vi "Focus Set Home.vi"(8 "error in (no error)":errorcluster, 10 "Motor (0:n-1)":i32, 11 "ArduinoFocus in":refnum<class "ArduinoFocus.lvclass">) -> (0 "error out":errorcluster, 3 "ArduinoFocus out":refnum<class "ArduinoFocus.lvclass">)   [LabVIEW 2022 SP3, in "ArduinoFocus.lvclass"]
uses:
  ArduinoFocus.lvclass
  ArduinoFocus.lvclass/ArduinoFocus.ctl
  Motor Control Driver/arduino Motor Control cluster Command.ctl
  Filter Wheel/Filter Wheel Arduino Control/FW Arduino Control.lvclass
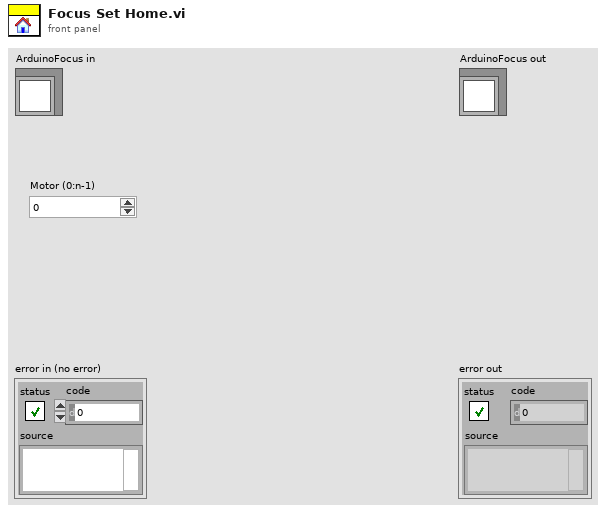
[diagram p1: front panel]
types:
  T1 = typedef "arduino Motor Control cluster Command.ctl" = cluster{"Direction":bool, "NUMBER OF  STEPS":u32, "SPEED STEPS/SEC":u16, "ACC/DECEL STEPS/SEC^2":u16, "EN/DIS?":bool}
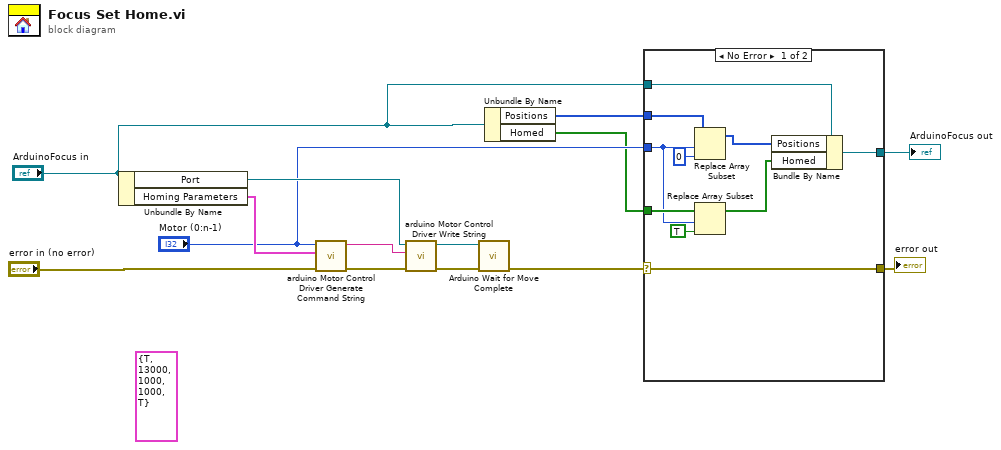
[diagram p0: block diagram]
diagram:
  (unwired) T1 {"Direction"=TRUE, "NUMBER OF  STEPS"=13000, "SPEED STEPS/SEC"=1000, "ACC/DECEL STEPS/SEC^2"=1000, "EN/DIS?"=TRUE} ("Command")
  n1 = Unbundle By Name("ArduinoFocus in") -> ("Port"=w12:refnum<visa-resource-name>, "Homing Parameters"=w8:T1)
  n2 = call "arduino Motor Control Driver Generate Command String.vi"("error in (no error)"="error in (no error)", "Command"=w8, "MOTOR NUMBER"="Motor (0:n-1)") -> ("error out"=w11:errorcluster, "Cmd String"=w13:string)  [unwired: 7 in]
  n3 = call "arduino Motor Control Driver Write String.vi"("error in (no error)"=w11, "String"=w13, "VISA resource name"=w12) -> ("error out"=w9:errorcluster, "VISA resource name out"=w10:refnum<visa-resource-name>)  [unwired: 7 in]
  n4 = call "Arduino Wait for Move Complete.vi"("error in (no error)"=w9, "reference"=w10) -> ("error out"=w5:errorcluster)  [unwired: 6 in, 3 out]
  n5 = Unbundle By Name("ArduinoFocus in") -> ("Positions"=w7:i32[], "Homed"=w4:bool[])
  n6 = case shown="No Error" w5 {
    selector: w5 -> [w15 w25]
    tunnel: w7 -> [w24 _]
    tunnel: "Motor (0:n-1)" -> [w21 _]
    tunnel: w4 -> [w22 _]
    tunnel: "ArduinoFocus in" -> [w19 w26]
    tunnel: [w16 w26] -> w2
    tunnel: [w15 w25] -> w1
    frame No Error {
      n7 = Replace Array Subset(array=w24, new element=0 ("new element/subarray"), index=w21) -> (w18:i32[])
      n8 = Replace Array Subset(array=w22, new element=TRUE ("new element/subarray"), index=w21) -> (w17:bool[])
      n9 = Bundle By Name(cluster=w19, "Positions"=w18, "Homed"=w17) -> (w16:refnum<class "ArduinoFocus.lvclass">)
    }
    frame Error {
    }
  }
  "error out" <- w1
  "ArduinoFocus out" <- w2
